vi "storeADC3BigFile.vi"(0 "chipNumber":string="99", 7 "Data Received":string, 11 "Test type":T1(ring)=enum."DAMIC_BUFF", 12 "current time":timestamp, 13 "comments":string) -> (15 "error out":errorcluster)   [LabVIEW 2014]
uses:
  Global/Global 1.vi
panel:
  out "typeTest":string
  out "justTime":string
  out "justDate":string
  out "outputFileName":string
  out "datetime":string
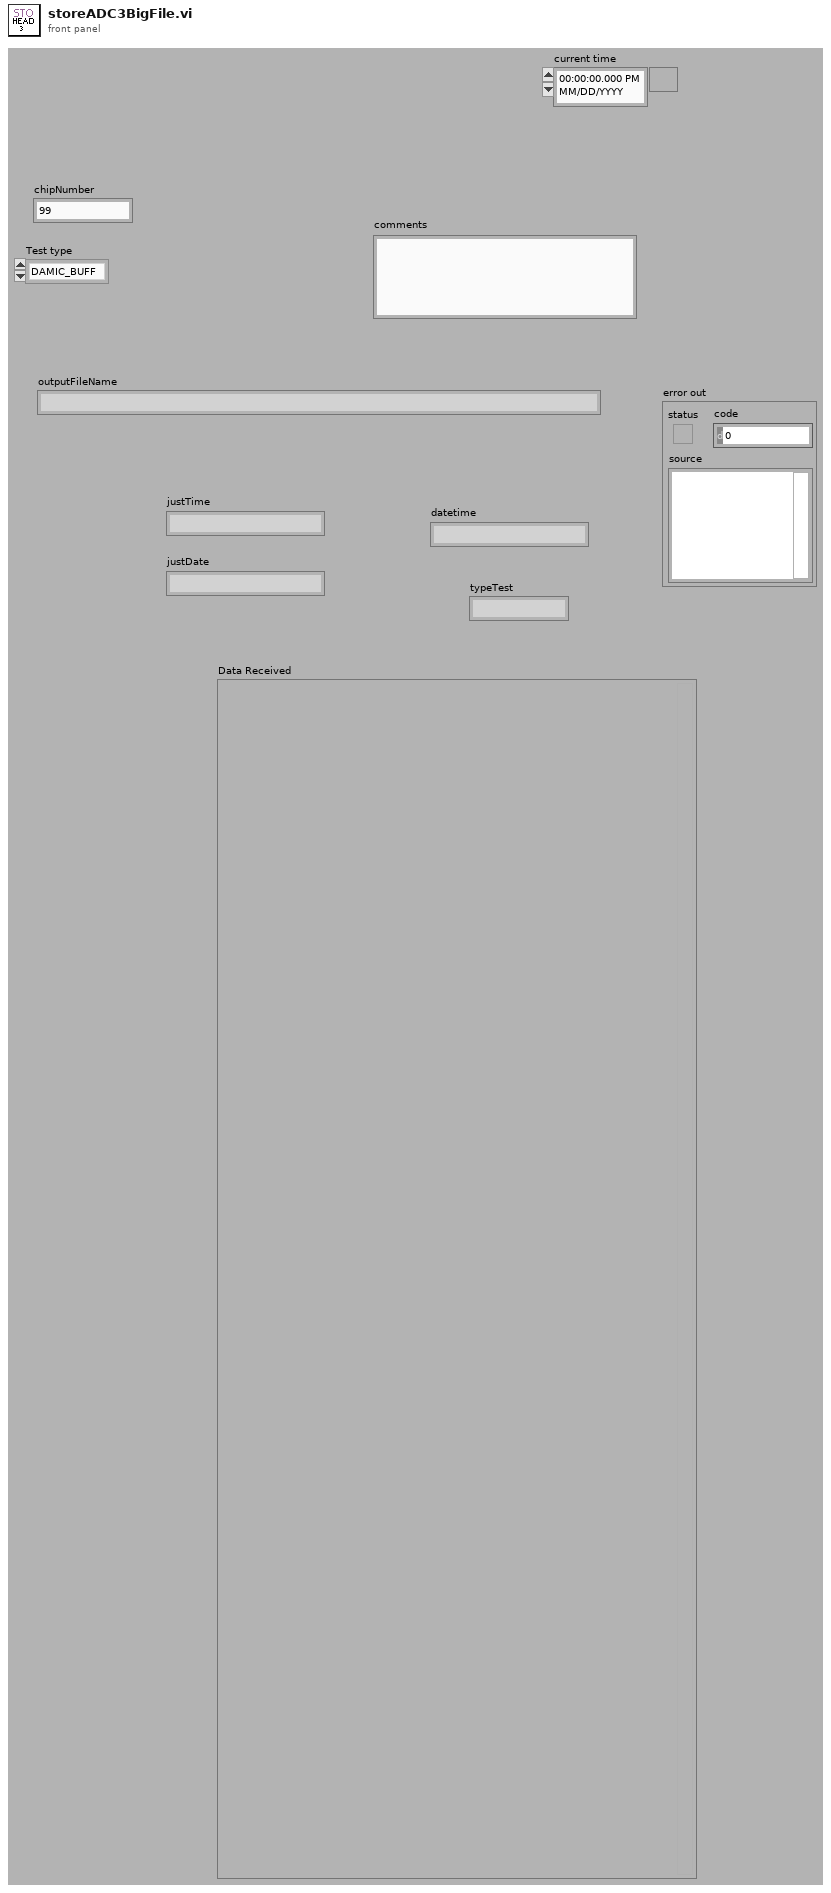
[diagram p1: front panel]
types:
  T1 = enum16{"DAMIC", "NOISE", "GAIN", "LINEAR18", "XTALK", "TEMP", "LINEAR16", "CONSO", "DAMIC_BUFF"}
  T2 = enum16{"open", "replace", "create", "open or create", "replace or create", "replace or create with confirmation"}
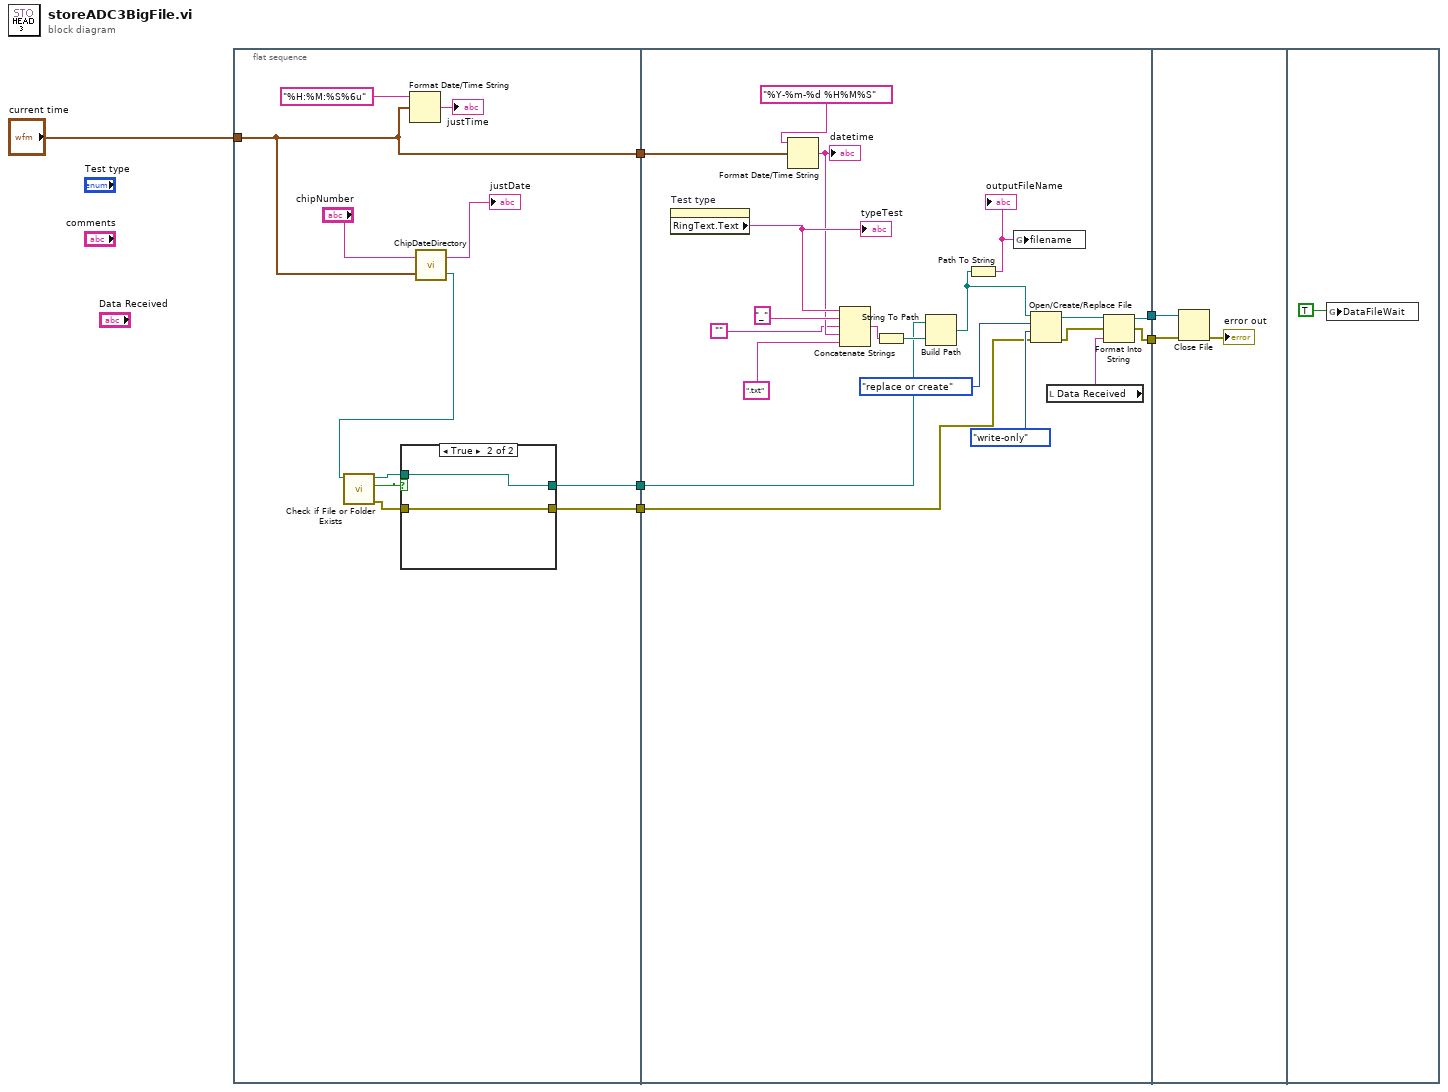
[diagram p0: block diagram]
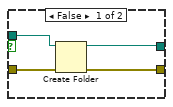
[diagram p2: hidden frame]
diagram:
  n1 = flat-sequence {
    tunnel: "current time" -> [w10]
    tunnel: [w10] -> w6
    tunnel: [w14] -> w5
    tunnel: [w11] -> w4
    tunnel: w6 -> [w39]
    tunnel: w5 -> [w25]
    tunnel: w4 -> [w35]
    tunnel: [w29] -> w2
    tunnel: [w27] -> w1
    tunnel: w2 -> [w45]
    tunnel: w1 -> [w46]
    frame #0 {
      n2 = Format Date/Time String(time format string (%c)="%H:%M:%S%6u", seconds (now)=w10) -> (date/time string=→"justTime":string)  [unwired: 1 in]
      n3 = call "ChipDateDirectory.vi"("time stamp"=w10, "chipNumber"="chipNumber") -> ("path"=w7:path, "justDate"=→"justDate":string)
      n4 = call <vilib>:"Check if File or Folder Exists.vi"("path"=w7) -> ("error out"=w12:errorcluster, "file or folder exists?"=w15:bool, "dup path"=w13:path)  [unwired: 1 in, 7 out]
      n5 = case shown="True" w15 {
        tunnel: [w20 w23] -> w14
        tunnel: w13 -> [w21 w23]
        tunnel: w12 -> [w19 w22]
        tunnel: [w18 w22] -> w11
        frame False {
          n6 = Create Folder(path (use dialog)=w21, error in=w19) -> (created path=w20:path, error out=w18:errorcluster)  [unwired: 2 out]
        }
        frame True {
        }
      }
    }
    frame #1 {
      n7 = property on="Test type" class="Enum (strict)"() -> ("RingText.Text"=w38:string)  [unwired: 2 in, 2 out]
      "typeTest" <- w38
      n8 = Format Date/Time String(time format string (%c)="%Y-%m-%d %H%M%S", seconds (now)=w39) -> (date/time string=w31:string)  [unwired: 1 in]
      "datetime" <- w31
      n9 = Concatenate Strings(w38, "_", "", w31, ".txt" ("string")) -> (w43:string)
      n10 = String To Path(string=w43) -> (path=w37:path)
      n11 = Build Path(base path=w25, name or relative path=w37) -> (appended path=w36:path)
      n12 = Path To String(path=w36) -> (string=w34:string)
      "outputFileName" <- w34
      n13 = global write "Global 1.vi" "filename"(w34) -> ()
      n14 = Open/Create/Replace File(file path (use dialog)=w36, error in=w35, operation (0:open)=T2."replace or create", access (0:read/write)=enum16{"read/write", "read-only", "write-only"}."write-only") -> (refnum out=w24:refnum<file>, error out=w28:errorcluster)  [unwired: 3 out]
      n15 = local read "Data Received"() -> (w26:string)
      n16 = Format Into String(initial string=w24, error in=w28, w26) -> (resulting string=w29:refnum<file>, error out=w27:errorcluster)  [unwired: 1 in]
    }
    frame #2 {
      n17 = Close File(refnum=w45, error in=w46) -> (error out=→"error out":errorcluster)  [unwired: 1 out]
    }
    frame #3 {
      n18 = global write "Global 1.vi" "DataFileWait"(TRUE) -> ()
    }
  }
